vi "Iteration.vi"(8 "error in (no error)":errorcluster, 10 "Process Value":dbl, 11 "PID in":refnum<class "PID.lvclass">) -> (0 "error out":errorcluster, 2 "Output":dbl, 3 "PID out":refnum<class "PID.lvclass">, 5 "Terms":T1)   [LabVIEW 2020, in "IG PID.lvlib" / "PID.lvclass"]
uses:
  PID.lvclass
  State.ctl
  PID.lvclass/PID.ctl
  IG PID.lvlib
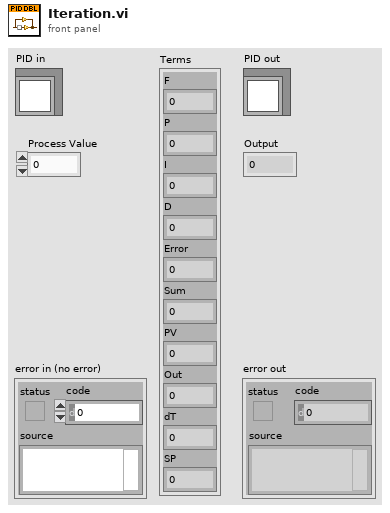
[diagram p1: front panel]
types:
  T1 = typedef "IG PID.lvlib/State.ctl" = cluster{"F":dbl, "P":dbl, "I":dbl, "D":dbl, "Error":dbl, "Sum":dbl, "PV":dbl, "Out":dbl, "dT":dbl, "SP":dbl}
  T2 = typedef "IG PID.lvlib/Output Range.ctl" = cluster{"Min":dbl, "Max":dbl}
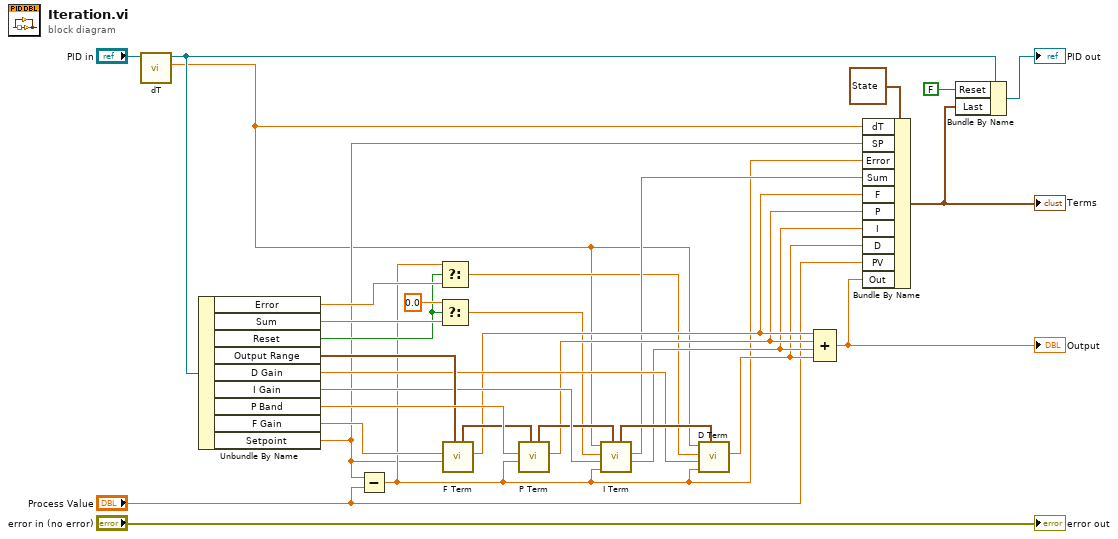
[diagram p0: block diagram]
diagram:
  n1 = call "dT.vi"("PID in"="PID in") -> ("dT"=w1:dbl, "PID out"=w24:refnum<class "PID.lvclass">)  [unwired: 8 in, 1 out]
  n2 = Unbundle By Name(w24) -> ("Error"=w12:dbl, "Sum"=w11:dbl, "Reset"=w9:bool, "Output Range"=w29:T2, "D Gain"=w21:dbl, "I Gain"=w27:dbl, "P Band"=w30:dbl, "F Gain"=w26:dbl, "Setpoint"=w2:dbl)
  n3 = Subtract(x=w2, y="Process Value") -> (x-y=w6:dbl)
  n4 = Select(t=w6, s=w9, f=w12) -> (s? t:f=w7:dbl)
  n5 = Select(t=0.0, s=w9, f=w11) -> (s? t:f=w8:dbl)
  n6 = call "F Term.vi"("Output Range"=w29, "Setpoint"=w2, "F Gain"=w26) -> ("Output"=w19:dbl, "Remaining Range"=w25:T2)  [unwired: 7 in]
  n7 = call "P Term.vi"("Output Range"=w25, "Error"=w6, "P Band"=w30) -> ("Output"=w18:dbl, "Remaining Range"=w23:T2)  [unwired: 7 in]
  n8 = call "I Term.vi"("Output Range"=w23, "Error"=w6, "I Gain"=w27, "Last Sum"=w8, "dT"=w1) -> ("Output"=w17:dbl, "Sum"=w15:dbl, "Remaining Range"=w22:T2)  [unwired: 4 in]
  n9 = call "D Term.vi"("Output Range"=w22, "Error"=w6, "D Gain"=w21, "Last Error"=w7, "dT"=w1) -> ("Output"=w16:dbl)  [unwired: 6 in]
  n10 = Compound Arithmetic op=ADD(w19, w18, w17, w16) -> (w3:dbl)
  "Output" <- w3
  n11 = Bundle By Name(cluster=T1 {"F"=0.0, "P"=0.0, "I"=0.0, "D"=0.0, "Error"=0.0, "Sum"=0.0, "PV"=0.0, "Out"=0.0, "dT"=0.0, "SP"=0.0} ("Outputs"), "dT"=w1, "SP"=w2, "Error"=w6, "Sum"=w15, "F"=w19, "P"=w18, "I"=w17, "D"=w16, "PV"="Process Value", "Out"=w3) -> (w5:T1)
  "Terms" <- w5
  n12 = Bundle By Name(cluster=w24, "Reset"=FALSE, "Last"=w5) -> (→"PID out":refnum<class "PID.lvclass">)
  "error out" <- "error in (no error)"
